vi "U6 Thermocouple Example.vi"(8 "error in":errorcluster) -> (0 "error out":errorcluster)   [LabVIEW 2021]
panel:
  in  "Ranges":u16[](array[ring])=[7, 7, 7, 7] items=["LJ_rgBIP10V", "LJ_rgBIP5V", "LJ_rgUNI5V", "LJ_rgUNI2P5V", "LJ_rgUNI1P25V", "LJ_rgBIP1V", "LJ_rgUNIP625V", "LJ_rgBIPP1V", "LJ_rgBIPP01V"]
  in  "-Ch":i32[](array[numeric])=[199, 199]
  in  "Gain":dbl=1.0 format="%.4f"
  in  "Cold Junction Sensor Offset [degK]":dbl format="%.4f"
  in  "Cold Junction Sensor Slope [degK/V]":dbl=1.0 format="%.4f"
  in  "Cold Junction Sensor Channel":i32=14
  out "Temperatures (Deg C)":dbl[](array[numeric]) format="%.2f"
  out "Cold Junction\nTemperature (Deg C)":dbl format="%.2f"
  in  "Offset Voltages":dbl[](array[numeric])=[0.0, 0.0] format="%.6f"
  in  "+Ch":i32[](array[numeric])=[0, 1]
  out "Raw Readings":dbl[](array[numeric]) format="%.6f"
  out "Error Message":string
  # "Uses the first found U6 over USB.\n\nAquires multiple analog input channels and performs a K type thermocouple conversion on them.  To\ndo an offset calibration, set the TCs near the U6 so they are at the same ambient temperature and thus\nthe measured voltage should be zero.  Allow time for everything to stabilize.  Then note the voltage\noffset in the \"Readings\" array, and enter this in the \"Offset\" array."
  # "If using an LJTIA (or other external amplifier) to amplify the\nthermocouple voltages, enter the gain here."
  # "The voltage from a thermocouple corresponds to the temperature\ndifference between one end and the other.  To determine the temp\nat the remote end, we must know the temperature at the local end.\nThe local end is called the cold junction, and in this case is\nthe U6 or CB37.  Enter the channel # from which to read the cold\njuntion temperature, and enter the slope/offset required to convert\nthat temperature to degrees K."
  # "Internal Sensor = 14"
  # "Internal=1, EI-1022=100, EI-1034=55.56"
  # "Internal=0, EI-1022=0, EI-1034=255.37"
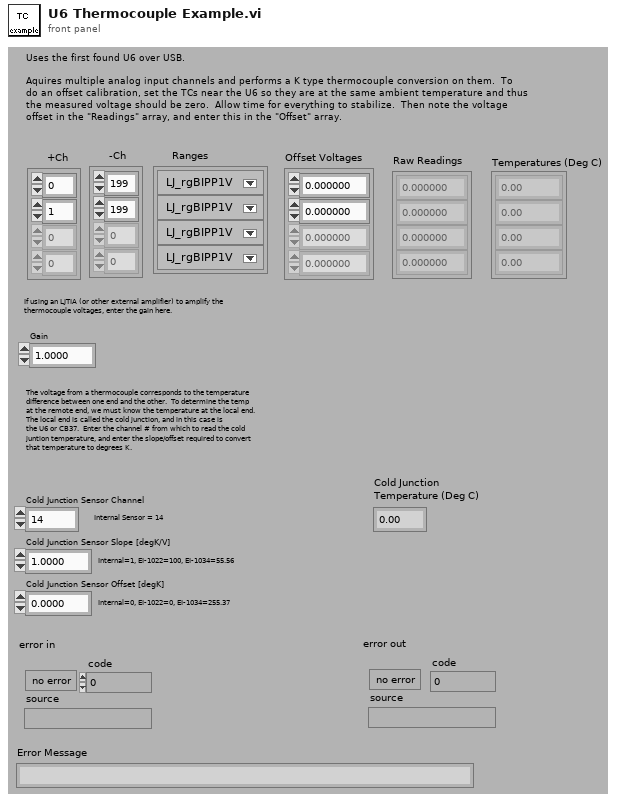
[diagram p1: front panel]
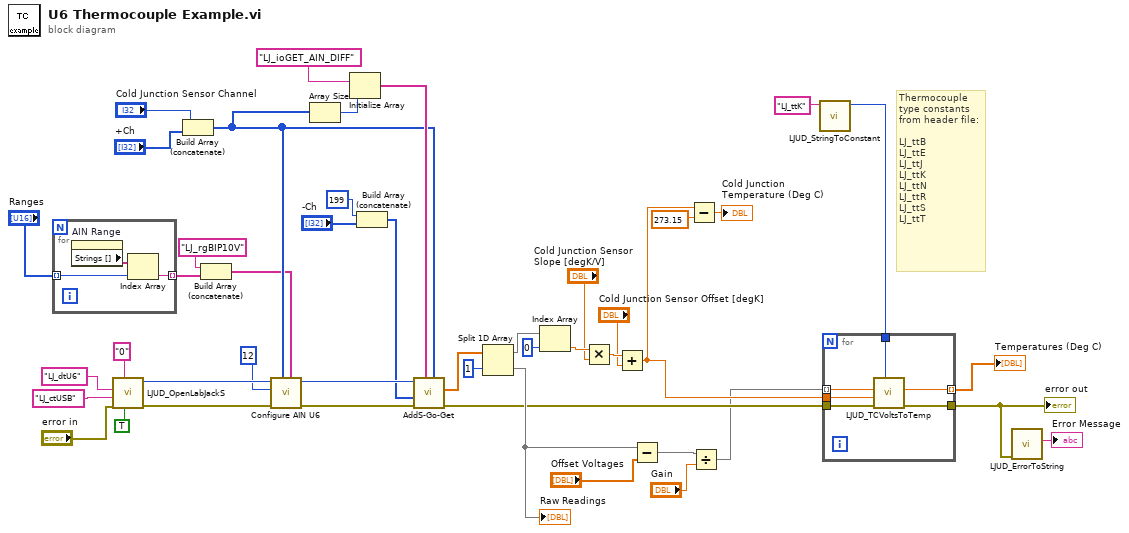
[diagram p0: block diagram]
diagram:
  # "Thermocouple\ntype constants\nfrom header file:\n\nLJ_ttB\nLJ_ttE\nLJ_ttJ\nLJ_ttK\nLJ_ttN\nLJ_ttR\nLJ_ttS\nLJ_ttT"
  n1 = for {
    tunnel: "Ranges" -> [w47] mode=indexing
    tunnel: [w46] -> w4 mode=indexing
    n2 = property on="AIN Range" class="Ring (strict)"() -> ("Strings []"=w48:string[])  [unwired: 2 in, 2 out]
    n3 = Index Array(array=w48, index=w47) -> (element=w46:string)
  }
  n4 = call "LJUD_OpenLabJackS.vi"("FirstFound"=TRUE, "Address"="0", "error in"="error in", "ConnectionType"="LJ_ctUSB", "DeviceType"="LJ_dtU6") -> ("error out"=w16:errorcluster, "Handle"=w13:i32)  [unwired: 4 in, 1 out]
  n5 = Build Array (concatenate)("Cold Junction Sensor Channel", "+Ch") -> (w3:i32[])
  n6 = Build Array (concatenate)("LJ_rgBIP10V" ("DeviceType"), w4) -> (w2:string[])
  n7 = call "Configure AIN U6.vi"("Ranges"=w2, "Positive Channels"=w3, "error in"=w16, "Resolution"=12, "Handle In"=w13) -> ("error out"=w15:errorcluster, "Handle Out"=w14:i32)  [unwired: 5 in]
  n8 = Array Size(array=w3) -> (size(s)=w11:i32)
  n9 = Initialize Array("LJ_ioGET_AIN_DIFF" ("IOType"), w11) -> (w40:string[])
  n10 = Build Array (concatenate)(199 ("Resolution"), "-Ch") -> (w5:i32[])
  n11 = call "AddS-Go-Get.vi"("Channels"=w3, "IOTypes"=w40, "error in"=w15, "x1"=w5, "Handle In"=w14) -> ("error out"=w22:errorcluster, "Values Read"=w35:dbl[])  [unwired: 4 in, 1 out]
  n12 = Split 1D Array(array=w35, index=1) -> (first subarray=w34:dbl[], second subarray=w23:dbl[])
  "Raw Readings" <- w23
  n13 = Index Array(array=w34, index=0 ("Index")) -> (element=w32:dbl)
  n14 = Multiply(x=w32, y="Cold Junction Sensor Slope [degK/V]") -> (x*y=w31:dbl)
  n15 = Add(x=w31, y="Cold Junction Sensor Offset [degK]") -> (x+y=w21:dbl)
  n16 = Subtract(x=w23, y="Offset Voltages") -> (x-y=w24:dbl[])
  n17 = Subtract(x=w21, y=273.15) -> (x-y=→"Cold Junction\nTemperature (Deg C)":dbl)
  n18 = Divide(x=w24, y="Gain") -> (x/y=w20:dbl[])
  n19 = call "LJUD_StringToConstant.vi"("String"="LJ_ttK") -> ("Constant Number"=w19:i32)  [unwired: 9 in, 1 out]
  n20 = for {
    tunnel: w22 -> [w54]
    tunnel: w21 -> [w53]
    tunnel: w20 -> [w52] mode=indexing
    tunnel: w19 -> [w51]
    tunnel: [w50] -> w18
    tunnel: [w49] -> w17 mode=indexing
    n21 = call "LJUD_TCVoltsToTemp.vi"("TCType"=w51, "error in"=w54, "CJTempK"=w53, "TCVolts"=w52) -> ("error out"=w50:errorcluster, "TCTempC"=w49:dbl)  [unwired: 4 in, 2 out]
  }
  "error out" <- w18
  "Temperatures (Deg C)" <- w17
  n22 = call "LJUD_ErrorToString.vi"("error in"=w18) -> ("String"=→"Error Message":string)  [unwired: 10 in]
